vi "Send Command.vi"(8 "error in (no error)":errorcluster, 9 "time out? (ms)":u32=50, 10 "operation":u32 format="%.0x", 11 "cluster of private data in":T1={"FPGA VI Reference"=refnum, "device index"=0, "screen size"=enum."8x1", "font size"=enum."5x8", "auto wrap"=FALSE, "alignment"=enum."None", "number of line"=enum."2 lines", "shift 0"=0, "entry mode 0"=enum."increment & no shift", "shift 1"=0, "entry mode 1"=enum."increment & no shift"}) -> (0 "error out":errorcluster, 2 "result":u32, 3 "cluster of private data out":T1={"FPGA VI Reference"=refnum, "device index"=0, "screen size"=enum."8x1", "font size"=enum."5x8", "auto wrap"=FALSE, "alignment"=enum."None", "number of line"=enum."2 lines", "shift 0"=0, "entry mode 0"=enum."increment & no shift", "shift 1"=0, "entry mode 1"=enum."increment & no shift"})   [LabVIEW 2017, in "HD44780.lvclass"]
uses:
  HD44780.lvclass
  <vilib>/Utility/error.llb/Error Cluster From Error Code.vi
  <vilib>/rvi/errors/niLvFpgaAdjustHostInterfaceError.vi
  <vilib>/rvi/interface/nirviReadWriteControl/nirviReadWriteControl.xnode
  Common/HD44780 Common.lvlib
  <vilib>/rvi/interface/Simulation/niFpgaSimulationCallBeginRW.vi
  NiFpgaLv.dll
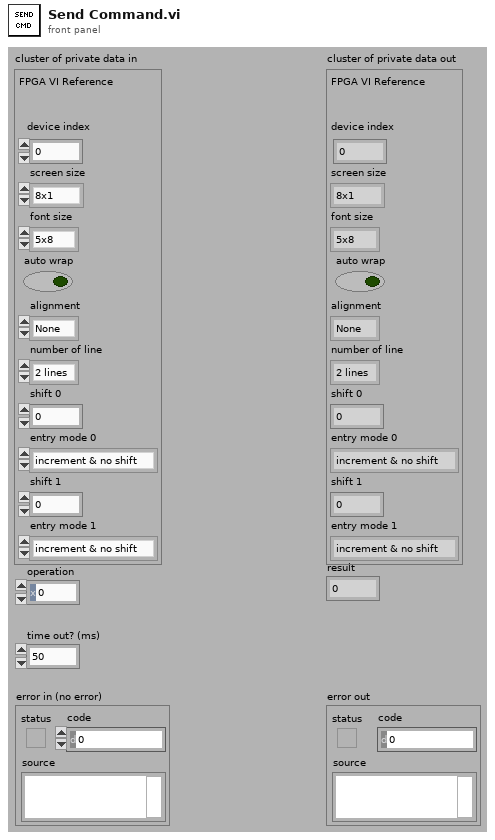
[diagram p1: front panel]
types:
  T1 = cluster{"FPGA VI Reference":refnum<k20>, "device index":i8, "screen size":enum8{"8x1", "8x2", "12x4", "16x1", "16x2", "16x4", "20x1", "20x2", "20x4", "24x1", "24x2", "40x2", "40x4"}, "font size":enum8{"5x8", "5x10"}, "auto wrap":bool, "alignment":enum16{"None", "Left", "Center", "Right"}, "number of line":enum8{"1 line", "2 lines"}, "shift 0":i8, "entry mode 0":enum8{"increment & no shift", "increment & shift", "decrement & no shift", "decrement & shift"}, "shift 1":i8, "entry mode 1":enum8{"increment & no shift", "increment & shift", "decrement & no shift", "decrement & shift"}}
  T2 = cluster{"device index (-1)":i8, "operation (0)":u32}
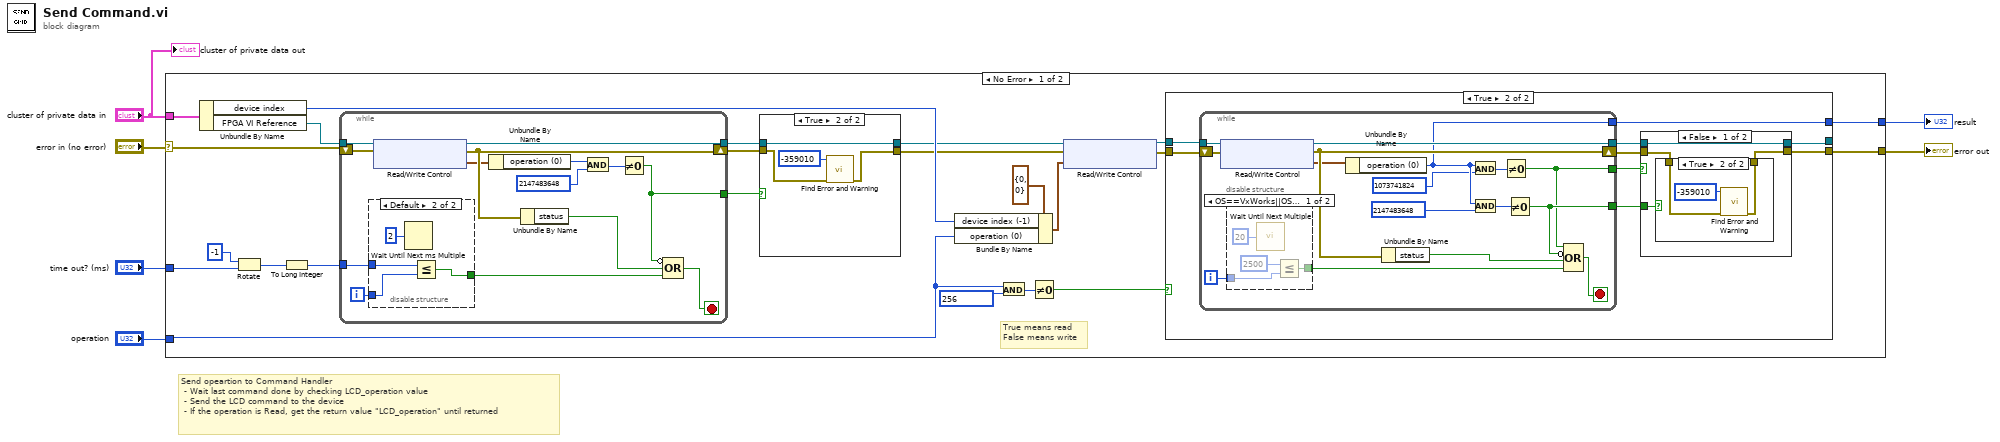
[diagram p0: block diagram]
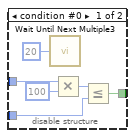
[diagram p2: hidden frame]
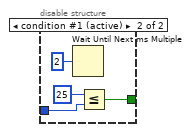
[diagram p4: hidden frame]
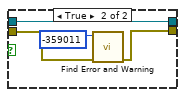
[diagram p6: hidden frame]
diagram:
  # "Send opeartion to Command Handler \n - Wait last command done by checking LCD_operation value \n - Send the LCD command to the device\n - If the operation is Read, get the return value \"LCD_operation\" until returned"
  n1 = case shown="No Error" "error in (no error)" {
    selector: "error in (no error)" -> [w26 w107]
    tunnel: [w16 w107] -> w6
    tunnel: "operation" -> [w22 _]
    tunnel: "cluster of private data in" -> [w27 _]
    tunnel: [w17 _] -> w2
    tunnel: "time out? (ms)" -> [w10 _]
    frame No Error {
      # "True means read\nFalse means write"
      n2 = Unbundle By Name(w27) -> ("device index"=w23:i8, "FPGA VI Reference"=w25:refnum<k20>)
      n3 = Rotate(1:w10, 2:i8 -1 ("y")) -> (0:w8:u32)
      n4 = To Long Integer(number=w8) -> (32bit integer=w7:i32)
      n5 = while {
        tunnel: w25 -> [w43]
        shift-right: [w41] -> w13
        shift-left: w26 -> [w42]
        tunnel: [w40] -> w12
        tunnel: [w38] -> w11
        tunnel: w7 -> [w33]
        i -> [w32]
        stop <- w30 stop-if-true
        n6 = disable-structure shown="Default" {
          disable-tunnel: w33 -> [w48 w52]
          disable-tunnel: w32 -> [w45 w51]
          disable-tunnel: [w44 w50] -> w31
          frame condition #0 {
            n7 = call "Wait Until Next Multiple3"("Count(uSec)"=u32 20) -> ()  [unwired: 1 out]
            n8 = Multiply(x=w48, y=100) -> (x*y=w46:i32)
            n9 = Less Or Equal?(x=w46, y=w45) -> (x <= y?=w44:bool)
          }
          frame condition #1 (active) {
            n10 = Wait Until Next ms Multiple(millisecond multiple=u32 2) -> ()  [unwired: 1 out]
            n11 = Less Or Equal?(x=w52, y=w51) -> (x <= y?=w50:bool)
          }
        }
        n12 = xnode "Read/Write Control"("FPGA VI Reference In"=w43, "error in"=w42) -> ("FPGA VI Reference Out"=w40:refnum<k20>, "error out"=w41:errorcluster, "LCD Command"=w37:T2)
        n13 = Unbundle By Name(w37) -> ("operation (0)"=w36:u32)
        n14 = Unbundle By Name(w41) -> ("status"=w39:bool)
        n15 = And(x=w36, y=u32 2147483648) -> (x .and. y?=w34:u32)
        n16 = Not Equal To 0?(x=w34) -> (x != 0?=w38:bool)
        n17 = Compound Arithmetic op=OR(invert w38, w39, w31) -> (w30:bool)
      }
      n18 = case shown="True" w11 {
        tunnel: [w102 w104] -> w20
        tunnel: w13 -> [w102 w105]
        tunnel: w12 -> [w101 w106]
        tunnel: [w101 w106] -> w21
        frame False {
        }
        frame True {
          n19 = call "Find Error and Warning.vi"("error in (no error)"=w105, "error code"=-359010) -> ("error out"=w104:errorcluster)  [unwired: 9 in]
        }
      }
      n20 = Bundle By Name(cluster=T2 {"device index (-1)"=0, "operation (0)"=0} ("LCD Command"), "device index (-1)"=w23, "operation (0)"=w22) -> (w19:T2)
      n21 = And(x=w22, y=u32 256) -> (x .and. y?=w15:u32)
      n22 = Not Equal To 0?(x=w15) -> (x != 0?=w24:bool)
      n23 = xnode "Read/Write Control"("FPGA VI Reference In"=w21, "error in"=w20, "LCD Command"=w19) -> ("FPGA VI Reference Out"=w29:refnum<k20>, "error out"=w28:errorcluster)
      n24 = case shown="True" w24 {
        tunnel: w29 -> [w55 w64]
        tunnel: w28 -> [w54 w63]
        tunnel: [w54 w62] -> w16
        tunnel: [w55 w61] -> _
        tunnel: [_ w56] -> w17
        frame False {
        }
        frame True {
          n25 = while {
            tunnel: w64 -> [w80]
            shift-right: [w78] -> w59
            shift-left: w63 -> [w79]
            tunnel: [w77] -> w60
            tunnel: [w75] -> w57
            tunnel: [w73] -> w58
            tunnel: [w72] -> w56
            i -> [w67]
            stop <- w65 stop-if-true
            n26 = xnode "Read/Write Control"("FPGA VI Reference In"=w80, "error in"=w79) -> ("FPGA VI Reference Out"=w77:refnum<k20>, "error out"=w78:errorcluster, "LCD Command"=w74:T2)
            n27 = disable-structure shown="OS==VxWorks||OS==PharLap" {
              disable-tunnel: w67 -> [w83 w85]
              disable-tunnel: [w82 w87] -> w66
              frame condition #0 {
                n28 = call "Wait Until Next Multiple"("Count(uSec)"=u32 20) -> ()  [unwired: 1 out]
                n29 = Less Or Equal?(x=2500 ("y"), y=w83) -> (x <= y?=w82:bool)
              }
              frame condition #1 (active) {
                n30 = Wait Until Next ms Multiple(millisecond multiple=u32 2) -> ()  [unwired: 1 out]
                n31 = Less Or Equal?(x=25 ("y"), y=w85) -> (x <= y?=w87:bool)
              }
            }
            n32 = Unbundle By Name(w74) -> ("operation (0)"=w72:u32)
            n33 = Unbundle By Name(w78) -> ("status"=w76:bool)
            n34 = And(x=w72, y=u32 1073741824) -> (x .and. y?=w71:u32)
            n35 = And(x=w72, y=u32 2147483648) -> (x .and. y?=w69:u32)
            n36 = Not Equal To 0?(x=w71) -> (x != 0?=w73:bool)
            n37 = Not Equal To 0?(x=w69) -> (x != 0?=w75:bool)
            n38 = Compound Arithmetic op=OR(w73, invert w75, w76, w66) -> (w65:bool)
          }
          n39 = case shown="False" w58 {
            tunnel: [w89 w98] -> w62
            tunnel: w59 -> [w90 w99]
            tunnel: w60 -> [w92 w100]
            tunnel: [w92 w100] -> w61
            tunnel: w57 -> [w91 _]
            frame False {
              n40 = case shown="True" w91 {
                tunnel: w90 -> [w93 w95]
                tunnel: [w93 w94] -> w89
                frame False {
                }
                frame True {
                  n41 = call "Find Error and Warning.vi"("error in (no error)"=w95, "error code"=-359010) -> ("error out"=w94:errorcluster)  [unwired: 9 in]
                }
              }
            }
            frame True {
              n42 = call "Find Error and Warning.vi"("error in (no error)"=w99, "error code"=-359011) -> ("error out"=w98:errorcluster)  [unwired: 9 in]
            }
          }
        }
      }
    }
    frame Error {
    }
  }
  "error out" <- w6
  "result" <- w2
  "cluster of private data out" <- "cluster of private data in"
